vi "ClsDownloadDeviceSpectrumsMultiChannelDevice.vi"(0 "Connection In":u32, 5 "Spectrum Type":i32, 7 "Start Channel Index":i32, 9 "Number of Channels":i32, 11 "error in (no error)":errorcluster) -> (4 "Connection Out":u32, 10 "Spectrums":i16[][](array[numeric]), 15 "error out":errorcluster)   [LabVIEW 2015]
doc: "Download Device Spectrums Multiple Channel:\n\nThis function is used for downloading spectrums from MPS/CLS devices. The required channels should be continuous. For example, if the client passes in \"10\" as the Start Channel Index, \"3\" as the number of Channels, spectrums of channel 10, 11, 12 will be downloaded from the device. All the spectrums have the same length. Note that the overall channel index of the device starts from 0.\n\nConnection In[Input]: the connection handle which is initially created by Open Connection subVI.\n\nSpectrum Type[Input]: Spectrum type: 0 for raw spectrum; 1 for processed spectrum in confocal mode; 2 for FFT spectrum in interferometric mode.\n\nStart Channel Index[Input]: the channel index of a section of continuous channels to get the spectrum. Note that the overall channel index of the device starts from 0.\n\nNumber of Channels[Input]: the number of channels to read the spectrums.\n\nSpectrums[Output]: the two dimensional array of requested spectrums. The first dimension is for different channels and the second dimension is for different pixels in a certain channel.\n\nConnection Out[Output]: the connection handle output which could be used for next subVI refering to the same connection."
uses:
  dependent dlls/CHRocodileDLL.dll
panel:
  out "Error Message 2":string
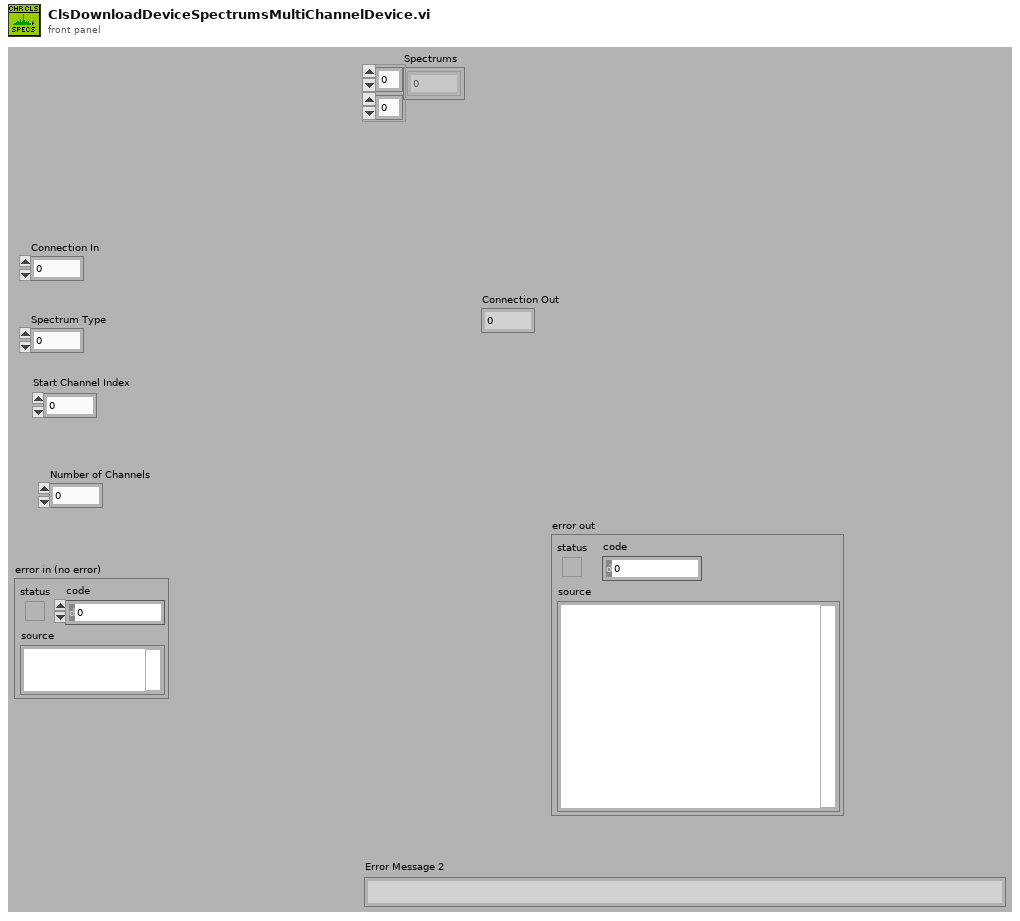
[diagram p1: front panel]
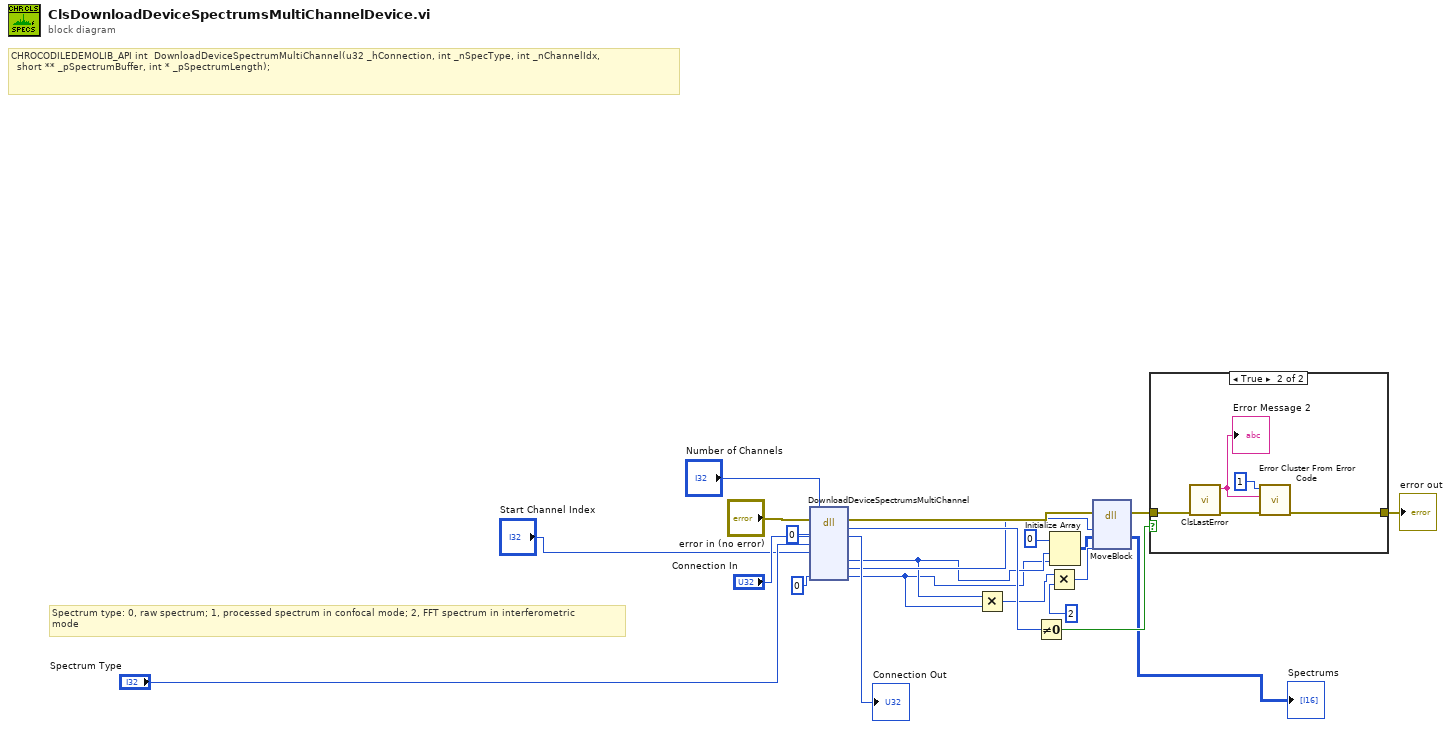
[diagram p0: block diagram]
diagram:
  # "Spectrum type: 0, raw spectrum; 1, processed spectrum in confocal mode; 2, FFT spectrum in interferometric\nmode"
  # "CHROCODILEDEMOLIB_API int  DownloadDeviceSpectrumMultiChannel(u32 _hConnection, int _nSpecType, int _nChannelIdx, \n\t\tshort ** _pSpectrumBuffer, int * _pSpectrumLength);"
  n1 = dll-call lib="C:/Users/privat/Documents/ADP-SLA/Drop Impact Teststand/dependent dlls/CHRocodileDLL.*" fn="DownloadDeviceSpectrumsMultiChannel"(error in="error in (no error)", "_hConnection"="Connection In", "_nSpecType"="Spectrum Type", "_nStartChannelIdx"="Start Channel Index", "_nChannelNumber"="Number of Channels", "_pSpectrumBuffer"=i64 0, "_pSingleSpectrumLength"=i64 0 ("_pSpectrumLength")) -> (error out=w11:errorcluster, "return type"=w17:i32, "_hConnection"=→"Connection Out":u32, "_nChannelNumber"=w4:i32, "_pSpectrumBuffer"=w9:i64, "_pSingleSpectrumLength"=w3:i64)  [unwired: 4 in, 1 out]
  n2 = Multiply(x=w4, y=w3) -> (x*y=w2:i64)
  n3 = Not Equal To 0?(x=w17) -> (x != 0?=w19:bool)
  n4 = Multiply(x=w2, y=2) -> (x*y=w13:i64)
  n5 = Initialize Array(i16 0, w4, w3) -> (w1:i16[][])
  n6 = dll-call lib="LabVIEW" fn="MoveBlock"(error in=w11, "Address(pointer)"=w9, "Destination"=w1, "Size"=w13) -> (error out=w10:errorcluster, "Destination"=→"Spectrums":i16[][])  [unwired: 5 in, 1 out]
  n7 = case shown="True" w19 {
    tunnel: [w23 w24] -> w18
    tunnel: w10 -> [w23 w27]
    frame False {
    }
    frame True {
      n8 = call "ClsLastError.vi"("error in (no error)"=w27) -> ("error out"=w26:errorcluster, "Error Message"=w25:string)  [unwired: 9 in]
      "Error Message 2" <- w25
      n9 = call <vilib>:"Error Cluster From Error Code.vi"("error in (no error)"=w26, "error message (\"\")"=w25, "error code (0)"=1) -> ("error out"=w24:errorcluster)  [unwired: 6 in]
    }
  }
  "error out" <- w18
